vi "Get AccessPDO.vi"(8 "Error In":errorcluster, 11 "reference in":refnum<class "OD Sub-Entry.lvclass">) -> (0 "Error Out":errorcluster, 2 "Access PDO":T1, 3 "reference out":refnum<class "OD Sub-Entry.lvclass">)   [LabVIEW 2024, in "Electronic Datasheet.lvlib" / "OD Sub-Entry.lvclass"]
uses:
  OD Sub-Entry.lvclass
  D:/git/EDS-File-Viewer/source/Core/OD Entry/OD Entry.lvclass
  OD Entry/OD Entry.lvclass
  OD Sub-Entry.lvclass/OD Sub-Entry.ctl
  Object Type.ctl
  Electronic Datasheet.lvlib
  c04c812d-fa3a-4f69-9024-5be920b84482.vi
  Access PDO.ctl
  PDO Mapping Type.ctl
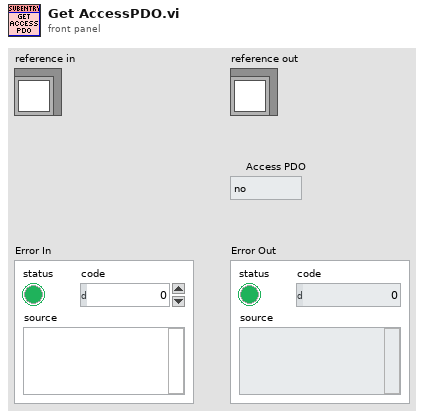
[diagram p1: front panel]
types:
  T1 = typedef "Electronic Datasheet.lvlib/Access PDO.ctl" = enum16{"no", "TPDO", "RPDO", "TPDO & RPDO"}
  T2 = enum16{"ro", "wo", "rw", "rwr", "rww", "const", "UNKNOWN"}
  T3 = typedef "Electronic Datasheet.lvlib/PDO Mapping Type.ctl" = enum16{"no", "optional", "RPDO", "TPDO", "UNKNOWN"}
  T4 = typedef "Electronic Datasheet.lvlib/Object Type.ctl" = u8
  T5 = typedef "Electronic Datasheet.lvlib/OD Sub-Entry.lvclass/ObjectAttributes.ctl" = cluster{"Parent":refnum<class "OD Entry.lvclass">}
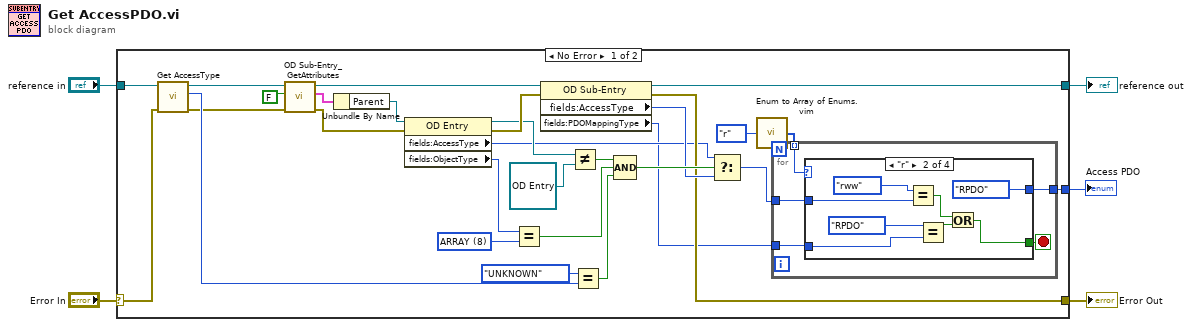
[diagram p0: block diagram]
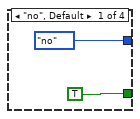
[diagram p2: hidden frame]
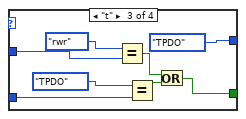
[diagram p3: hidden frame]
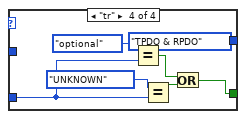
[diagram p4: hidden frame]
diagram:
  n1 = case shown="No Error" "Error In" {
    selector: "Error In" -> [w28 w66]
    tunnel: [w11 w66] -> w4
    tunnel: [w14 w65] -> w2
    tunnel: "reference in" -> [w34 w65]
    tunnel: [w7 _] -> w1
    frame No Error {
      w22 = T4 8 items=["NULL"=0, "DOMAIN"=2, "DEFTYPE"=5, "DEFSTRUCT"=6, "VAR"=7, "ARRAY"=8, "RECORD"=9] ("ObjectType")
      n2 = call "Get AccessType.vi"("Error In"=w28, "reference in"=w34) -> ("Error Out"=w24:errorcluster, "AccessType"=w27:T2, "reference out"=w23:refnum<class "OD Sub-Entry.lvclass">)  [unwired: 7 in]
      n3 = call "OD Sub-Entry_GetAttributes.vi"("Error In"=w24, "OnlyGetDvrReference(False)"=FALSE, "reference in"=w23) -> ("Error Out"=w20:errorcluster, "Data"=w31:T5, "reference out"=w33:refnum<class "OD Sub-Entry.lvclass">)  [unwired: 5 in, 1 out]
      n4 = Unbundle By Name(w31) -> ("Parent"=w10:refnum<class "OD Entry.lvclass">)
      n5 = property class="OD Entry"(reference=w10, error in=w20) -> (reference out=w18:refnum<class "OD Entry.lvclass">, error out=w19:errorcluster, "fields:AccessType"=w8:T2, "fields:ObjectType"=w9:T4)
      n6 = Equal?(x=w9, y=w22) -> (x = y?=w21:bool)
      n7 = property class="OD Sub-Entry"(reference=w33, error in=w19) -> (reference out=w14:refnum<class "OD Sub-Entry.lvclass">, error out=w11:errorcluster, "fields:AccessType"=w12:T2, "fields:PDOMappingType"=w6:T3)
      n8 = Not Equal?(x=w18, y=refnum<class "OD Entry.lvclass"> refnum) -> (x != y?=w29:bool)
      n9 = Equal?(x=T2."UNKNOWN", y=w27) -> (x = y?=w25:bool)
      n10 = Compound Arithmetic op=AND(w29, w21, w25) -> (w15:bool)
      n11 = Select(t=w8, s=w15, f=w12) -> (s? t:f=w13:T2)
      n12 = call "Enum to Array of Enums.vim"("enum"=enum16{"r", "t", "tr", "no"}."r") -> ("array of enums"=w17:enum16{"r", "t", "tr", "no"}[])
      n13 = for {
        tunnel: w17 -> [w39] mode=indexing
        tunnel: w13 -> [w38]
        tunnel: w6 -> [w37]
        tunnel: [w35] -> w7
        stop <- w36 stop-if-true
        n14 = case shown="\"r\"" w39 {
          tunnel: w38 -> [_ w43 w54 _]
          tunnel: w37 -> [_ w44 w52 w60]
          tunnel: [TRUE w47 w55 w62] -> w36
          tunnel: [Access_PDO."no" ("Access PDO") Access_PDO."RPDO" ("Access PDO") Access_PDO."TPDO" ("Access PDO") Access_PDO."TPDO & RPDO" ("Access PDO")] -> w35
          frame "no", Default {
          }
          frame "r" {
            n15 = Equal?(x=T2."rww" ("y"), y=w43) -> (x = y?=w49:bool)
            n16 = Equal?(x=PDO_Mapping_Type."RPDO" ("y"), y=w44) -> (x = y?=w48:bool)
            n17 = Or(x=w49, y=w48) -> (x .or. y?=w47:bool)
          }
          frame "t" {
            n18 = Equal?(x=T2."rwr" ("y"), y=w54) -> (x = y?=w57:bool)
            n19 = Equal?(x=PDO_Mapping_Type."TPDO" ("y"), y=w52) -> (x = y?=w56:bool)
            n20 = Or(x=w57, y=w56) -> (x .or. y?=w55:bool)
          }
          frame "tr" {
            n21 = Equal?(x=PDO_Mapping_Type."optional", y=w60) -> (x = y?=w64:bool)
            n22 = Equal?(x=PDO_Mapping_Type."UNKNOWN", y=w60) -> (x = y?=w63:bool)
            n23 = Or(x=w64, y=w63) -> (x .or. y?=w62:bool)
          }
        }
      }
    }
    frame Error {
    }
  }
  "Error Out" <- w4
  "reference out" <- w2
  "Access PDO" <- w1
